vi "template_WiFi_SmartConfig.vi"   [LabVIEW 2014]
doc: "is a desing template VI for WiFi with Smart Config feature."
uses:
  QwaveSys_ESP8266/QwaveSys_ESP8266.lvlib
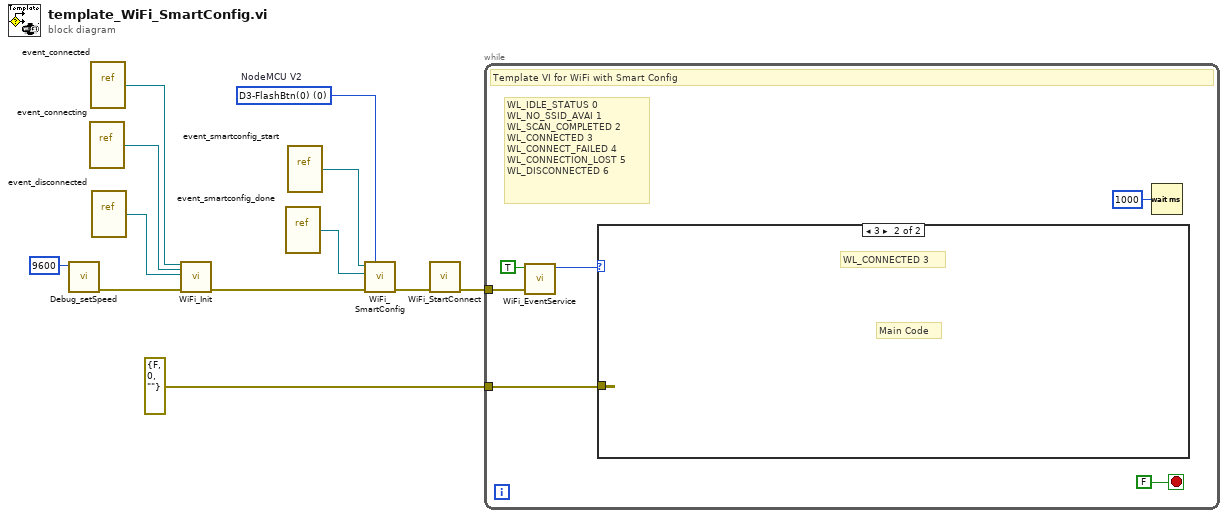
[diagram p0: block diagram]
diagram:
  w4 = u8 0 items=["D0-(LED)-(16)"=16, "D1-SCL(5)"=5, "D2-SDA(4)"=4, "D3-FlashBtn(0)"=0, "D4-(2)"=2, "D5-SCK(14)"=14, "D6-MISO(12)"=12, "D7-MOSI(13)"=13, "D8-SS(15)"=15, "D9-TX(3)"=3, "D10-RX(1)"=1]  # NodeMCU V2
  n1 = call "Debug_setSpeed.vi"("Speed"=u32 9600) -> ("error out"=w2:errorcluster)  [unwired: 10 in]
  n2 = vi-ref "event_connecting.vi"() -> (w9:refnum<vi>)
  n3 = vi-ref "event_connected.vi"() -> (w8:refnum<vi>)
  n4 = vi-ref "event_disconnected.vi"() -> (w7:refnum<vi>)
  n5 = call "WiFi_Init.vi"("connected"=w8, "connecting"=w9, "disconnected"=w7, "error in (no error)"=w2) -> ("error out"=w12:errorcluster)  [unwired: 11 in]
  n6 = vi-ref "event_smartconfig_done.vi"() -> (w5:refnum<vi>)
  n7 = vi-ref "event_smartconfig_start.vi"() -> (w6:refnum<vi>)
  n8 = call "WiFi_SmartConfig.vi"("Smart Config Enter Pin"=w4, "error in (no error)"=w12, "smartconfig_done"=w5, "smartconfig_start"=w6) -> ("error out"=w11:errorcluster)  [unwired: 7 in]
  n9 = call "WiFi_StartConnect.vi"("error in (no error)"=w11) -> ("error out"=w10:errorcluster)  [unwired: 10 in]
  n10 = while {
    tunnel: w10 -> [w17]
    tunnel: errorcluster {"status"=FALSE, "code"=0, "source"=""} ("error out") -> [w13]
    stop <- FALSE stop-if-true
    # "WL_IDLE_STATUS\t0\nWL_NO_SSID_AVAI\t1\nWL_SCAN_COMPLETED\t2\nWL_CONNECTED\t3\nWL_CONNECT_FAILED\t4\nWL_CONNECTION_LOST\t5\nWL_DISCONNECTED\t6"
    # "Template VI for WiFi with Smart Config"
    n11 = call "WiFi_EventService.vi"("error in (no error)"=w17, "wait for connected (True)"=TRUE) -> ("Status"=w14:u16)  [unwired: 8 in, 1 out]
    n12 = case shown="3" w14 {
      tunnel: w13 -> [_ _]
      frame 0, Default {
        # "DISCONNECTED or default status"
      }
      frame 3 {
        # "WL_CONNECTED\t3"
        # "Main Code"
      }
    }
    n13 = Wait (ms)(milliseconds to wait=u32 1000) -> ()  [unwired: 1 out]
  }
